vi "Display.vi"(8 "error in":errorcluster, 11 "Timeout Two Button in":refnum<class "Gif - Timeout Two Button.lvclass">) -> (0 "error out":errorcluster, 3 "Timeout Two Button out":refnum<class "Gif - Timeout Two Button.lvclass">)   [LabVIEW 2021, in "Gif - Timeout Two Button.lvclass"]
doc: "This vi displays the custom image two button timeout popup.\n\n<b>Code Developed By:</b>\nDaniel Coons\nTechnology Service Corporation\n1983 S Liberty Drive\nBloomington, IN 47403\nPhone: 812 558-7100\ndaniel.coons@tsc.com\nwww.tsc.com"
uses:
  Gif - Timeout Two Button.lvclass
  C:/Program Files/National Instruments/LabVIEW 2024/vi.lib/addons/_TSC/TSC Pop-Up/Popup/Popup.lvclass
  C:/Development/tsc-pop-up-gif/GIF Parent.lvclass
  <vilib>/Utility/miscctls.llb/LVPositionTypeDef.ctl
  Gif - Timeout Two Button.lvclass/Gif - Timeout Two Button.ctl
  <vilib>/addons/_TSC/TSC Pop-Up/Popup/Popup.lvclass/Popup.ctl
  GIF Parent.lvclass/GIF Parent.ctl
  <vilib>/addons/_TSC/TSC Pop-Up/Popup/Data Member Access/Read Theme.vi
  Read Delays.vi
  Read Gif Images.vi
  <vilib>/addons/_TSC/TSC Pop-Up/Theme/Theme.lvclass
  <vilib>/addons/_TSC/TSC Pop-Up/Popup/Popup.lvclass
  user32.dll
panel:
  in  "closer":bool
  out "header":bool
  out "count":string
  in  "n-text":bool
  in  "y-text":bool
  out "2D Picture":picture
  out "Message":string
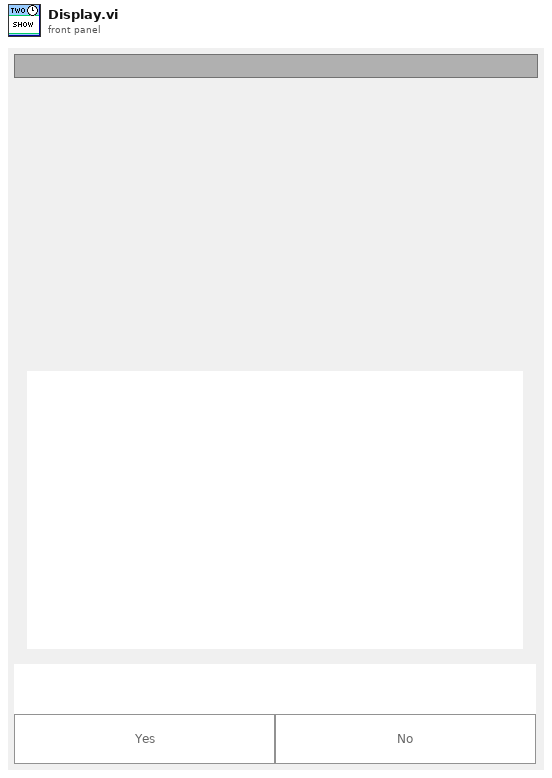
[diagram p1: front panel]
types:
  T1 = typedef "LVPositionTypeDef.ctl" = cluster{"Left":i32, "Top":i32}
  T2 = typedef "LVPoint32TypeDef.ctl" = cluster{"Horizontal":i32, "Vertical":i32}
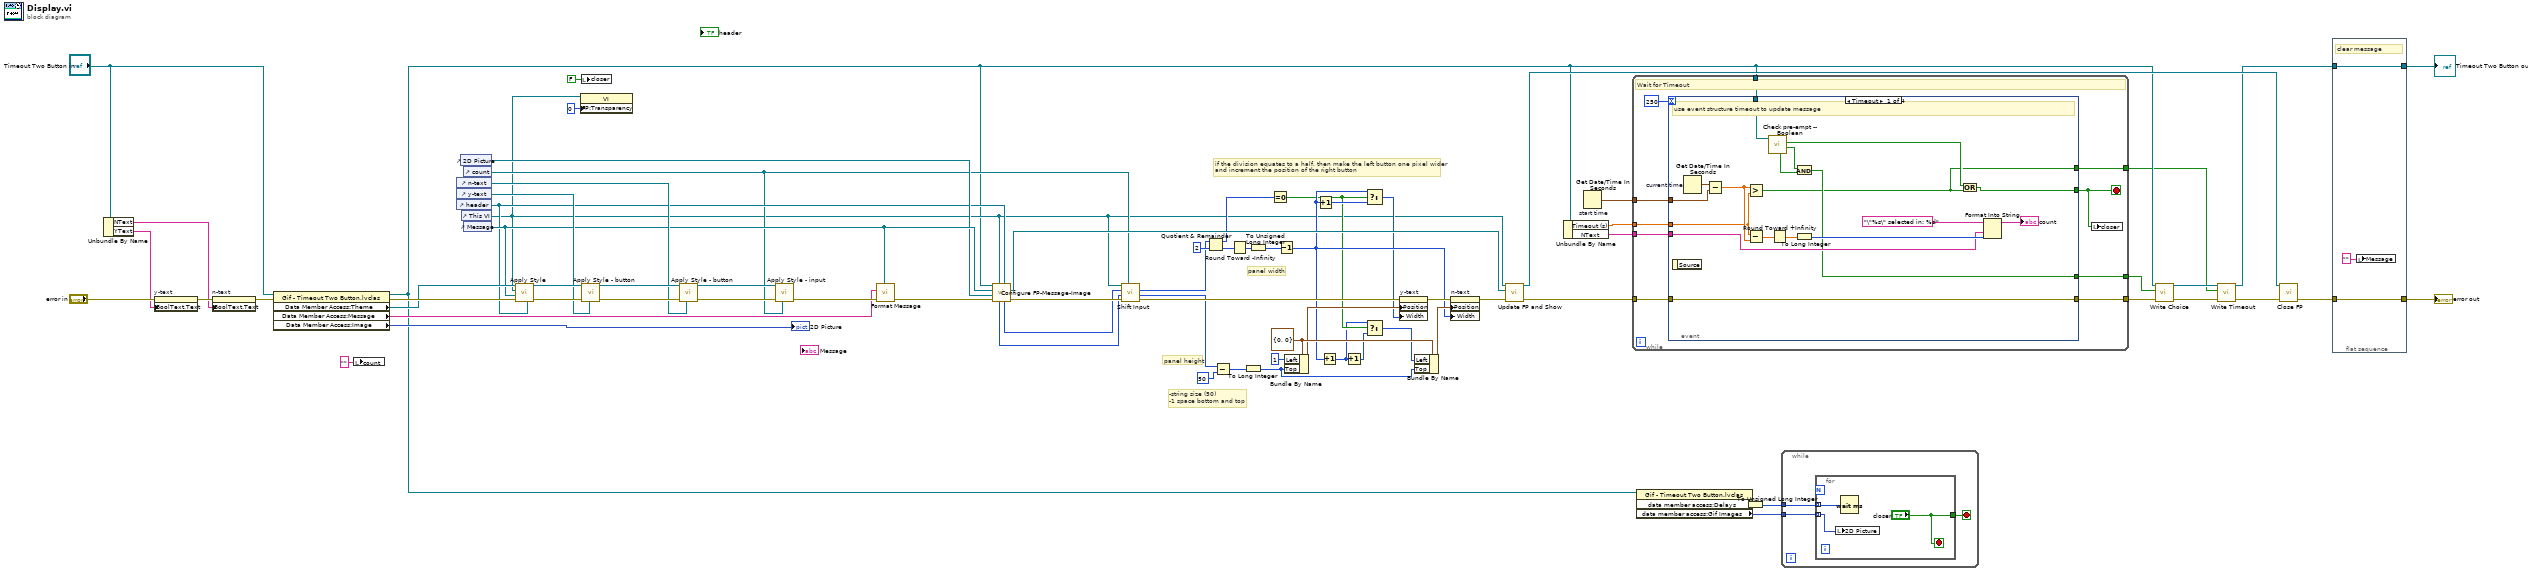
[diagram p0: block diagram]
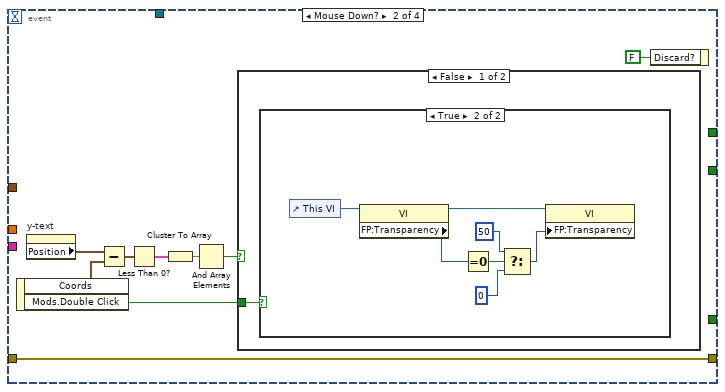
[diagram p2: hidden frame]
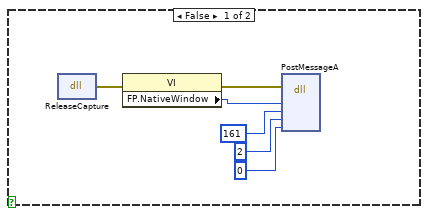
[diagram p3: hidden frame]
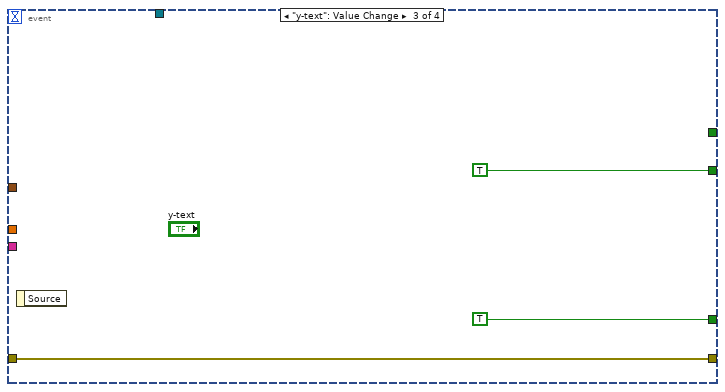
[diagram p5: hidden frame]
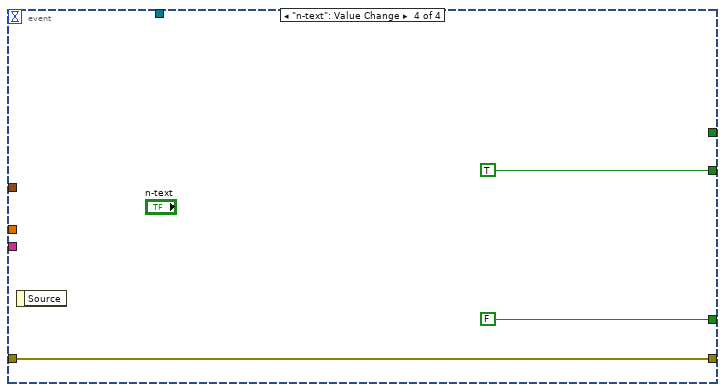
[diagram p6: hidden frame]
diagram:
  w44 = T1 {"Left"=0, "Top"=0} ("Position")
  # "if the division equates to a half, then make the left button one pixel wider \nand increment the position of the right button"
  # "-string size (50)\n-1 space bottom and top"
  # "panel width"
  # "panel height"
  n1 = Unbundle By Name("Timeout Two Button in") -> ("NText"=w70:string, "YText"=w72:string)
  n2 = property on="y-text" class="Bool"(error in="error in", "BoolText.Text"=w72) -> (error out=w73:errorcluster)  [unwired: 1 in, 1 out]
  n3 = property on="n-text" class="Bool"(error in=w73, "BoolText.Text"=w70) -> (error out=w71:errorcluster)  [unwired: 1 in, 1 out]
  n4 = property class="Gif - Timeout Two Button.lvclas"(reference="Timeout Two Button in", error in=w71) -> (reference out=w6:refnum<class "Gif - Timeout Two Button.lvclass">, error out=w57:errorcluster, "Data Member Access:Theme"=w55:refnum<class "Theme.lvclass">, "Data Member Access:Message"=w46:string, "Data Member Access:Image"=→"2D Picture":picture)
  n5 = local write "count"("" ("count")) -> ()
  n6 = control-ref of="n-text"() -> (w49:refnum<vi>)
  n7 = control-ref of="y-text"() -> (w50:refnum<vi>)
  n8 = control-ref of="header"() -> (w27:refnum<vi>)
  n9 = control-ref of="2D Picture"() -> (w28:refnum<vi>)
  n10 = control-ref of="This VI"() -> (w11:refnum<vi>)
  n11 = control-ref of="count"() -> (w24:refnum<vi>)
  n12 = control-ref of="Message"() -> (w29:refnum<vi>)
  n13 = call <vilib>:"Apply Style.vi"("header ref"=w27, "error in (no error)"=w57, "message ref"=w29, "pop up ref"=w11, "Theme in"=w55) -> ("error out"=w56:errorcluster, "Theme out"=w51:refnum<class "Theme.lvclass">)  [unwired: 5 in]
  n14 = property class="VI"(reference=w11, "FP:Transparency"=u8 0 ("Front Panel Window:Transparency")) -> ()  [unwired: 1 in, 2 out]
  n15 = local write "closer"(FALSE ("closer")) -> ()
  n16 = call <vilib>:"Apply Style - button.vi"("button ref"=w50, "error in (no error)"=w56, "Theme in"=w51) -> ("error out"=w54:errorcluster, "Theme out"=w52:refnum<class "Theme.lvclass">)  [unwired: 7 in]
  n17 = call <vilib>:"Apply Style - button.vi"("button ref"=w49, "error in (no error)"=w54, "Theme in"=w52) -> ("error out"=w53:errorcluster, "Theme out"=w47:refnum<class "Theme.lvclass">)  [unwired: 7 in]
  n18 = call <vilib>:"Apply Style - input.vi"("input ref"=w24, "error in (no error)"=w53, "Theme in"=w47) -> ("error out"=w48:errorcluster)  [unwired: 7 in, 1 out]
  n19 = call <vilib>:"Format Message.vi"("formatted string"=w29, "error in"=w48, "String Input"=w46) -> ("error out"=w31:errorcluster)  [unwired: 7 in, 1 out]
  n20 = call <vilib>:"Configure FP-Message-Image.vi"("header ref"=w27, "Pop Up ref"=w11, "error in (no error)"=w31, "Image ref"=w28, "Message ref"=w29, "Popup in"=w6) -> ("error out"=w32:errorcluster, "Panel Ref"=w26:refnum<vi>, "Panel Width"=w23:i32, "Panel Height"=w21:i32)  [unwired: 1 in, 1 out]
  n21 = call <vilib>:"Shift Input.vi"("Control"=w24, "Error In"=w32, "Panel Height"=w21, "Panel Width"=w23, "Pop Up ref"=w11) -> ("Error Out"=w25:errorcluster, "Panel Height out"=w20:i32, "Panel Width out"=w22:i32)  [unwired: 4 in]
  n22 = Quotient & Remainder(x=w22, y=2) -> (x-y*floor(x/y)=w19:i32, floor(x/y)=w36:i32)
  n23 = Subtract(x=w20, y=50 ("value")) -> (x-y=w39:i32)
  n24 = Round Toward -Infinity(1:w36) -> (0:w33:i32)
  n25 = To Long Integer(number=w39) -> (32bit integer=w42:i32)
  n26 = To Unsigned Long Integer(number=w33) -> (unsigned 32bit integer=w34:u32)
  n27 = Equal To 0?(x=w19) -> (x = 0?=w15:bool)
  n28 = Decrement(x=w34) -> (x-1=w18:u32)
  n29 = Bundle By Name(cluster=w44, "Left"=1, "Top"=w42) -> (w40:T1)
  n30 = Increment(x=w18) -> (x+1=w17:u32)
  n31 = Increment(x=w18) -> (x+1=w14:u32)
  n32 = Increment(x=w14) -> (x+1=w13:u32)
  n33 = Select(t=w18, s=w15, f=w17) -> (s? t:f=w16:u32)
  n34 = Select(t=w14, s=w15, f=w13) -> (s? t:f=w12:u32)
  n35 = property on="y-text" class="Bool"(error in=w25, "Position"=w40, "Width"=w16) -> (error out=w41:errorcluster)  [unwired: 1 in, 1 out]
  n36 = Bundle By Name(cluster=w44, "Left"=w12, "Top"=w42) -> (w43:T1)
  n37 = property on="n-text" class="Bool"(error in=w41, "Position"=w43, "Width"=w18) -> (error out=w30:errorcluster)  [unwired: 1 in, 1 out]
  n38 = call <vilib>:"Update FP and Show.vi"("error in (no error)"=w30, "Panel Ref"=w26, "VI in"=w11) -> ("error out"=w69:errorcluster, "VI out"=w59:refnum<vi>)  [unwired: 7 in]
  n39 = Unbundle By Name(w6) -> ("Timeout (s)"=w67:dbl, "NText"=w66:string)
  n40 = Get Date/Time In Seconds "start time"() -> (seconds since 1Jan1904=w68:timestamp)
  n41 = while {
    tunnel: [w81] -> w65
    tunnel: w69 -> [w82]
    tunnel: w68 -> [w85]
    tunnel: w67 -> [w84]
    tunnel: w66 -> [w80]
    tunnel: [w79] -> w64
    tunnel: w6 -> [w78]
    tunnel: [w76] -> w1
    stop <- w77 stop-if-true
    # "Wait for Timeout"
    n42 = event shown="[0] Timeout" {
      selector: _ -> [_ _ _ _]
      dyn-events: _ -> [_ _ _ _]
      timeout: 250 -> [_ _ _ _]
      tunnel: w85 -> [w103 _ _ _]
      tunnel: [w93 _ TRUE TRUE] -> w77
      tunnel: w84 -> [w99 _ _ _]
      tunnel: w82 -> [w97 w111 w129 w132]
      tunnel: [w97 w111 w129 w132] -> w81
      tunnel: w80 -> [w95 _ _ _]
      tunnel: [w89 _ TRUE FALSE] -> w79
      tunnel: w78 -> [w94 _ _ _]
      tunnel: [w86 _ _ _] -> w76
      event Timeout {
        # "use event structure timeout to update message"
        n43 = event-data() -> ()  [unwired: 1 in, 1 out]
        n44 = Get Date/Time In Seconds "current time"() -> (seconds since 1Jan1904=w102:timestamp)
        n45 = Subtract(x=w102, y=w103) -> (x-y=w101:dbl)
        n46 = Greater?(x=w101, y=w99) -> (0:w86:bool)
        n47 = Subtract(x=w99, y=w101) -> (x-y=w100:dbl)
        n48 = call <vilib>:"Check pre-empt -- Boolean.vi"("_Popup in"=w94) -> ("Value?"=w91:bool, "Pre-empted?"=w92:bool, "Type Match?"=w90:bool)  [unwired: 7 in, 1 out]
        n49 = Round Toward +Infinity(x=w100) -> (ceil(x): smallest int >= x=w87:dbl)
        n50 = And(x=w91, y=w90) -> (x .and. y?=w89:bool)
        n51 = To Long Integer(number=w87) -> (32bit integer=w96:i32)
        n52 = Or(x=w92, y=w86) -> (x .or. y?=w93:bool)
        n53 = Format Into String(format string="\"%s\" selected in: %d", w95, w96) -> (resulting string=→"count":string)  [unwired: 2 in, 1 out]
      }
      event Mouse Down? {
        n54 = event-data() -> ("Coords"=w104:T2, "Mods.Double Click"=w105:bool)  [unwired: 1 in]
        n55 = property on="y-text" class="Bool"() -> ("Position"=w110:T1)  [unwired: 2 in, 2 out]
        n56 = Subtract(x=w110, y=w104) -> (x-y=w109:T1)
        n57 = Less Than 0?(x=w109) -> (x < 0?=w108:cluster{"Left":bool, "Top":bool})
        n58 = Cluster To Array(cluster=w108) -> (array=w107:bool[])
        n59 = And Array Elements(Boolean array=w107) -> (logical AND=w106:bool)
        n60 = case shown="False" w106 {
          tunnel: w105 -> [w113 _]
          frame False {
            n61 = case shown="True" w113 {
              frame False {
                n62 = dll-call lib="user32.dll" fn="ReleaseCapture"() -> (error out=w117:errorcluster)  [unwired: 4 in, 1 out]
                n63 = property class="VI"(error in=w117) -> (error out=w118:errorcluster, "FP.NativeWindow"=w119:u64)  [unwired: 1 in, 1 out]
                n64 = dll-call lib="user32.dll" fn="PostMessageA"(error in=w118, "hWnd"=w119, "Msg"=161, "wParam"=2, "lParam"=0) -> ()  [unwired: 7 in, 2 out]
              }
              frame True {
                n65 = control-ref of="This VI"() -> (w126:refnum<vi>)
                n66 = property class="VI"(reference=w126) -> (reference out=w124:refnum<vi>, "FP:Transparency"=w125:u8)  [unwired: 1 in, 1 out]
                n67 = Equal To 0?(x=w125) -> (x = 0?=w123:bool)
                n68 = Select(t=u8 50, s=w123, f=u8 0) -> (s? t:f=w122:u8)
                n69 = property class="VI"(reference=w124, "FP:Transparency"=w122) -> ()  [unwired: 1 in, 2 out]
              }
            }
          }
          frame True {
          }
        }
        n70 = event-data("Discard?"=FALSE) -> ()  [unwired: 1 in, 1 out]
      }
      event "y-text": Value Change {
        n71 = event-data() -> ()  [unwired: 1 in, 1 out]
      }
      event "n-text": Value Change {
        n72 = event-data() -> ()  [unwired: 1 in, 1 out]
      }
    }
    n73 = local write "closer"(w77) -> ()
  }
  n74 = property class="Gif - Timeout Two Button.lvclas"(reference=w6) -> ("data member access:Delays"=w9:i32[], "data member access:Gif Images"=w8:picture[])  [unwired: 1 in, 2 out]
  n75 = To Unsigned Long Integer(number=w9) -> (unsigned 32bit integer=w7:u32[])
  n76 = while {
    tunnel: w7 -> [w134]
    tunnel: w8 -> [w133]
    stop <- w135 stop-if-true
    n77 = for {
      tunnel: ["closer"] -> w135
      tunnel: w134 -> [w137] mode=indexing
      tunnel: w133 -> [w136] mode=indexing
      stop <- "closer" stop-if-true
      n78 = local write "2D Picture"(w136) -> ()
      n79 = Wait (ms)(milliseconds to wait=w137) -> ()  [unwired: 1 out]
    }
  }
  n80 = call-dynamic "Write Choice.vi"("error in (no error)"=w65, "Choice"=w64, "_Popup in"=w6) -> ("error out"=w62:errorcluster, "_Popup out"=w3:refnum<class "Gif - Timeout Two Button.lvclass">)  [unwired: 7 in]
  n81 = call <vilib>:"Write Timeout.vi"("error in (no error)"=w62, "Timeout?"=w1, "Popup in"=w3) -> ("error out"=w4:errorcluster, "Popup out"=w2:refnum<class "Gif - Timeout Two Button.lvclass">)  [unwired: 7 in]
  n82 = call <vilib>:"Close FP.vi"("error in (no error)"=w4, "VI in"=w59) -> ("error out"=w63:errorcluster)  [unwired: 9 in]
  n83 = flat-sequence {
    tunnel: w63 -> [w141]
    tunnel: [w141] -> w61
    tunnel: w2 -> [w140]
    tunnel: [w140] -> w60
    frame #0 {
      # "clear message"
      n84 = local write "Message"("" ("Message")) -> ()
    }
  }
  "error out" <- w61
  "Timeout Two Button out" <- w60
